vi "TEST - Set Control Value {Variant}.vi"(8 "error in (no error)":errorcluster) -> (0 "error out":errorcluster, 2 "pass":bool)   [LabVIEW 2020]
uses:
  <userlib>/_OpenG.lib/lvdata/lvdata.llb/Type Descriptor Enumeration__ogtk.ctl
  <userlib>/_OpenG.lib/error/error.llb/openg_error.lvlib
  <userlib>/_OpenG.lib/lvdata/lvdata.llb/openg_variant.lvlib
panel:
  in  "MyBoolean":bool
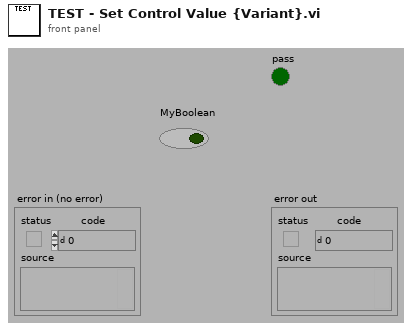
[diagram p1: front panel]
types:
  T1 = typedef "openg_variant.lvlib/Type Descriptor Enumeration__ogtk.ctl" = enum8{"<Null>", "I8", "I16", "I32", "I64", "U8", "U16", "U32", "U64", "SGL", "DBL", "EXT", "CSG", "CDB", "CXT", "0x0F", "0x10", "0x11", "0x12", "0x13", "0x14", "Enum U8", "Enum U16", "Enum U32", "Enum U64", "SGL PQ", "DBL PQ", "EXT PQ", "CSG PQ", "CDB PQ", "CXT PQ", "0x1F", "0x20", "Boolean", "0x22", "0x23", "0x24", "0x25", "0x26", "0x27", "0x28", "0x29", "0x2A", "0x2B", "0x2C", "0x2D", "0x2E", "0x2F", "String", "0x31", "Path", "Pict", "0x34", "0x35", "0x36", "DAQ", "0x38", "0x39", "0x3A", "0x3B", "0x3C", "0x3D", "0x3E", "0x3F", "Array", "0x41", "0x42", "0x43", "0x44", "0x45", "0x46", "0x47", "0x48", "0x49", "0x4A", "0x4B", "0x4C", "0x4D", "0x4E", "0x4F", "Cluster", "0x51", "0x52", "Variant", "Waveform", "0x55", "0x56", "0x57", "0x58", "0x59", "0x5A", "0x5B", "0x5C", "0x5D", "0x5E", "Fixed Point", "0x60", "0x61", "0x62", "0x63", "0x64", "0x65", "0x66", "0x67", "0x68", "0x69", "0x6A", "0x6B", "0x6C", "0x6D", "0x6E", "0x6F", "Refnum", "0x71", "0x72", "Set Collection", "Map Collection"}
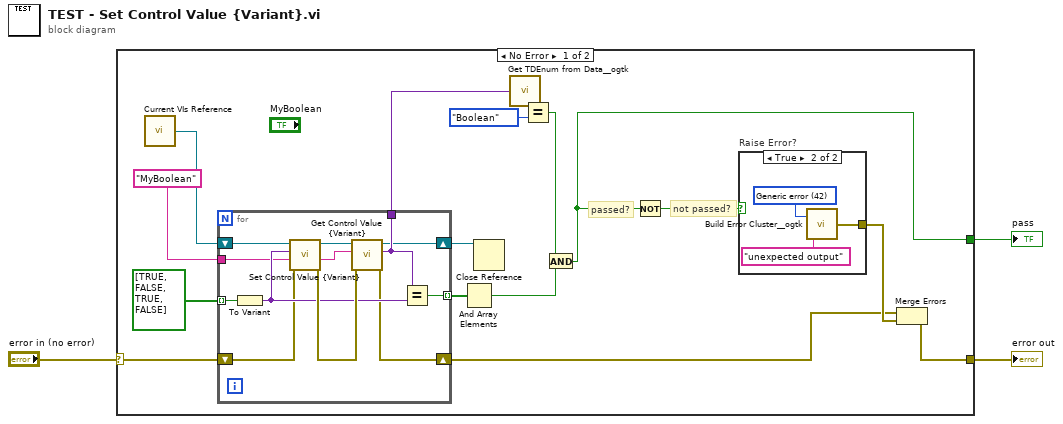
[diagram p0: block diagram]
diagram:
  n1 = case shown="No Error" "error in (no error)" {
    selector: "error in (no error)" -> [w7 w34]
    tunnel: [w4 _] -> w3
    tunnel: [w19 w34] -> w1
    frame No Error {
      # "not passed?"
      # "passed?"
      n2 = call "Current VIs Reference.vi"() -> ("Current VI's reference"=w10:refnum<vi>)  [unwired: 5 in]
      n3 = for {
        tunnel: bool[] [TRUE, FALSE, TRUE, FALSE] -> [w28] mode=indexing
        tunnel: [w27] -> w14
        tunnel: "MyBoolean" ("Name") -> [w25]
        tunnel: [w24] -> w9 mode=indexing
        shift-right: [w23] -> w11
        shift-left: w10 -> [w22]
        shift-right: [w21] -> w8
        shift-left: w7 -> [w20]
        n4 = To Variant(anything=w28) -> (Variant=w26:variant)
        n5 = call "Set Control Value {Variant}.vi"("error in (no error)"=w20, "Control Name (\"\": use variant name)"=w25, "Value"=w26, "VI Refnum"=w22) -> ("error out"=w30:errorcluster, "VI Refnum dup"=w29:refnum<vi>)  [unwired: 6 in]
        n6 = call "Get Control Value {Variant}.vi"("error in (no error)"=w30, "Control Name"=w25, "VI Refnum"=w29) -> ("error out"=w21:errorcluster, "Value"=w27:variant, "VI Refnum dup"=w23:refnum<vi>)  [unwired: 6 in]
        n7 = Equal?(x=w27, y=w26) -> (x = y?=w24:bool)
      }
      n8 = And Array Elements(Boolean array=w9) -> (logical AND=w6:bool)
      n9 = Close Reference(reference=w11) -> ()  [unwired: 1 in, 1 out]
      n10 = call <userlib>:"Get TDEnum from Data__ogtk.vi"("Data"=w14) -> ("Type Descriptor Enumeration"=w15:T1)  [unwired: 4 in]
      n11 = Equal?(x=w15, y=Type_Descriptor_Enumeration__ogtk."Boolean" ("Type Descriptor Enumeration")) -> (x = y?=w5:bool)
      n12 = And(x=w5, y=w6) -> (x .and. y?=w4:bool)
      n13 = Not(x=w4) -> (.not. x?=w17:bool)
      n14 = case "Raise Error?" shown="True" w17 {
        tunnel: [_ w31] -> w18
        frame False {
        }
        frame True {
          w32 = 42 items=["No error", "Argument error", "Memory is full", "Out of zone", "End of file", "File already open", "Generic file I/O error", "File not found", "File permission error", "Disk is full", "Duplicate path", "Too many files open", "System feature not enabled", "Resource file not found", "Cannot add resource", "Resource not found", "Image not found", "Image memory error", "Pen does not exist", "Config type invalid", "Config token not found", "Config parse error", "Config memory error", "Bad external code format", "Bad external code offset", "External code not present", "Null window", "Destroy window error", "Null menu", "Print aborted", "Bad print record", "Print driver error", "Windows error during printing", "Memory error during printing", "Print dialog error", "Generic print error", "Invalid device refnum", "Device not found", "Device parameter error", "Device unit error", "Cannot open device", "Device call aborted", "Generic error", "Cancelled by user", "Object ID too low", "Object ID too high", "Object not in heap", "Unknown heap", "Unknown object (invalid DefProc)", "Unknown object (DefProc not in table)", "Message out of range", "Invalid (null) method", "Unknown message", "Manager call not supported", "Bad address", "Network operation in progress", "Network operation timed out", "Connection is busy", "Network attribute not supported", "Network error", "Address in use", "System out of memory", "Connection aborted", "Connection refused", "Not connected", "Already connected", "Connection closed", "Initialization error (interapplication manager)", "Bad occurrence", "Wait on unbound occurrence handler", "Occurrence queue overflow", "Datalog type conflict", "Unused", "Unrecognized type (interapplication manager)", "Memory corrupt", "Failed to make temporary DLL", "Old CIN version", "Drag socket not found", "Failed to load drop-object", "Failed to register OLE object", "Failed to release OLE object", "Format specifier type mismatch", "Unknown format specifier", "Too few format specifiers", "Too many format specifiers", "Scan failed", "Newer CIN version", "Error converting to variant", "Runtime menu error", "Password tampered", "Variant attribute not found", "Incompatible variant data type", "Event data is not available", "Event Store is not present", "Occurrence is not found", "Event Queue is not created", "Event info is not available", "Refnum passed is NULL", "Error retrieving Class GUID", "Error retrieving CoClass GUID", "Error retrieving TypeLib GUID.", "Bad built application magic bytes.", "Specific driver is different from the specific driver associated with the Logical Name.", "There is no session opened to the class driver.", "Max Error", "MAX - Error with config objects", "MAX - Error loading configuration", "MAX - Group not supported"]
          n15 = call <userlib>:"Build Error Cluster__ogtk.vi"("String to Prepend to source (\"\")"="unexpected output" ("String to Prepend to source (\"\")"), "code"=w32) -> ("error out"=w31:errorcluster)
        }
      }
      n16 = Merge Errors(w8, w18) -> (w19:errorcluster)
    }
    frame Error {
    }
  }
  "pass" <- w3
  "error out" <- w1
